vi "Check Decoupling.vi"(1 "Valve package":T1, 2 "Current Pos":dbl, 3 "Moving Dir (-1, 0, 1)":i32, 4 "Checked-in?":bool) -> (0 "Sample Car left in Valve (decoupled)?":bool)   [LabVIEW 2016, in "Hardware.lvlib" / "VacuumLine.lvlib" / "VacuumLine.lvclass"]
uses:
  <userlib>/Common Components/Hardware/Abstract System/VacuumLine/VacuumLine/VacuumLine.lvclass
  <userlib>/Common Components/Hardware/Abstract System/VacuumLine/VacuumLine/Valve Complex.ctl
  <userlib>/Common Components/Hardware/Abstract System/VacuumLine/VacuumLine/Logic Cluster.ctl
panel:
  # "Pin#"
  # "Location"
  # "Tolerance"
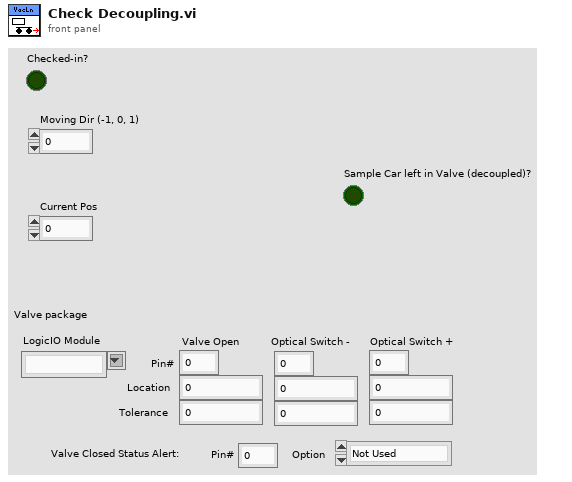
[diagram p1: front panel]
types:
  T1 = typedef "Hardware.lvlib/VacuumLine.lvlib/VacuumLine.lvclass/Valve Complex.ctl" = cluster{"LogicIO Module":string, "Valve Open":T2, "Optical Switch -":T2, "Optical Switch +":T2, "Valve Closed Status Alert":cluster{"Pin#":u8, "Option":enum16{"Not Used", "Normally Closed"}}}
  T2 = typedef "Hardware.lvlib/VacuumLine.lvlib/VacuumLine.lvclass/Logic Cluster.ctl" = cluster{"Pin#":u8, "Location":dbl, "Tolerance":dbl}
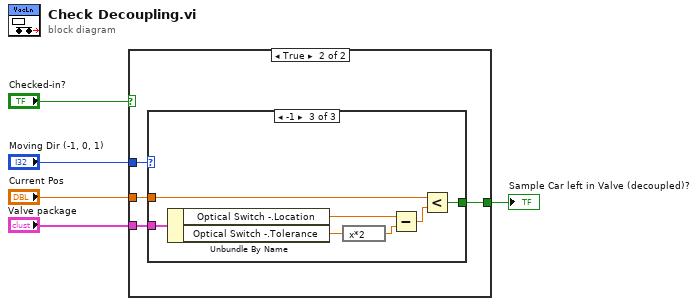
[diagram p0: block diagram]
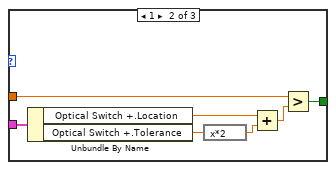
[diagram p4: hidden frame]
diagram:
  n1 = case shown="True" "Checked-in?" {
    tunnel: "Moving Dir (-1, 0, 1)" -> [_ w9]
    tunnel: "Valve package" -> [_ w6]
    tunnel: "Current Pos" -> [_ w8]
    tunnel: [_ w7] -> w2
    frame False {
    }
    frame True {
      n2 = case shown="-1" w9 {
        tunnel: w8 -> [_ w16 w23]
        tunnel: [_ w15 w22] -> w7
        tunnel: w6 -> [_ w12 w20]
        frame 0, Default {
        }
        frame 1 {
          n3 = Unbundle By Name(w12) -> ("Optical Switch +.Location"=w13:dbl, "Optical Switch +.Tolerance"=w14:dbl)
          n4 = expression code="x*2"(w14) -> (w10:dbl)
          n5 = Add(x=w13, y=w10) -> (x+y=w11:dbl)
          n6 = Greater?(x=w16, y=w11) -> (0:w15:bool)
        }
        frame -1 {
          n7 = Unbundle By Name(w20) -> ("Optical Switch -.Location"=w18:dbl, "Optical Switch -.Tolerance"=w21:dbl)
          n8 = expression code="x*2"(w21) -> (w17:dbl)
          n9 = Subtract(x=w18, y=w17) -> (x-y=w19:dbl)
          n10 = Less?(x=w23, y=w19) -> (x < y?=w22:bool)
        }
      }
    }
  }
  "Sample Car left in Valve (decoupled)?" <- w2
